vi "getCategoryNamesArray.vi"(8 "error in (no error)":errorcluster, 11 "CategoryList in":refnum<class "CategoryList.lvclass">) -> (0 "error out":errorcluster, 2 "Category Names":string[](array[string]), 3 "CategoryList out":refnum<class "CategoryList.lvclass">)   [LabVIEW 2018, in "CategoryList.lvclass"]
uses:
  CategoryList.lvclass
  CategoryList.lvclass/CategoryList.ctl
  Category/Category.lvclass
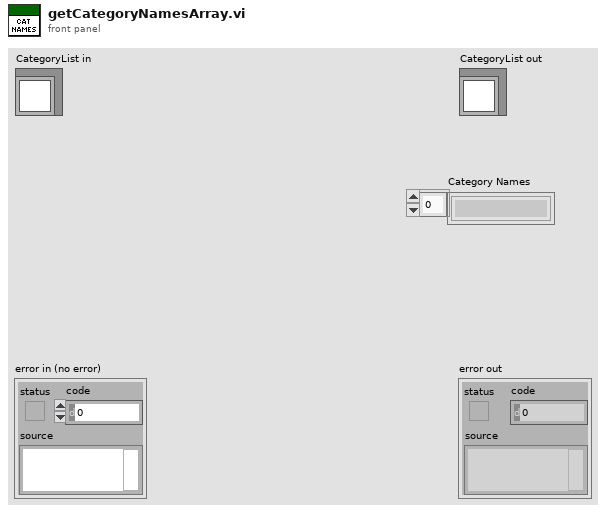
[diagram p1: front panel]
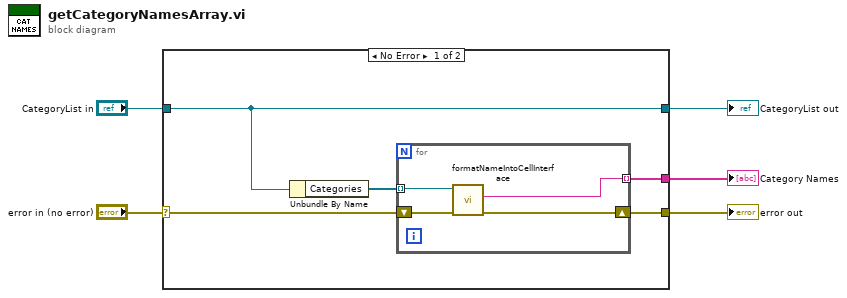
[diagram p0: block diagram]
diagram:
  n1 = case shown="No Error" "error in (no error)" {
    selector: "error in (no error)" -> [w7 w16]
    tunnel: [w6 w16] -> w4
    tunnel: [w10 w15] -> w2
    tunnel: "CategoryList in" -> [w10 w15]
    tunnel: [w8 _] -> w1
    frame No Error {
      n2 = Unbundle By Name(w10) -> ("Categories"=w9:refnum<class "Category.lvclass">[])
      n3 = for {
        tunnel: w9 -> [w14] mode=indexing
        tunnel: [w11] -> w8 mode=indexing
        shift-right: [w12] -> w6
        shift-left: w7 -> [w13]
        n4 = call "formatNameIntoCellInterface.vi"("error in (no error)"=w13, "Category in"=w14) -> ("error out"=w12:errorcluster, "Name"=w11:string)  [unwired: 7 in, 1 out]
      }
    }
    frame Error {
    }
  }
  "error out" <- w4
  "CategoryList out" <- w2
  "Category Names" <- w1
